vi "Round Timestamp to Tenth of Second.vi"(1 "Time Stamp (now)":timestamp) -> (0 "Time Stamp":timestamp)   [LabVIEW 2011]
doc: "Rounds Timestamp to the nearest tenth of a second.\n\nReturns current time if input is unwired.\n\nVersion 1.0 - 03/07/2013\n\nPhaeron, Inc.\nwww.phaeron.com\ninfo@phaeron.com"
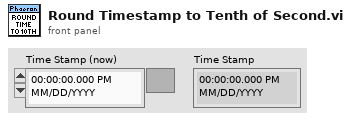
[diagram p1: front panel]
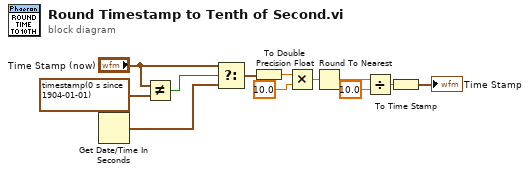
[diagram p0: block diagram]
diagram:
  n1 = Get Date/Time In Seconds() -> (seconds since 1Jan1904=w5:timestamp)
  n2 = Not Equal?(x="Time Stamp (now)", y=timestamp(0 s since 1904-01-01) ("Time Stamp")) -> (x != y?=w4:bool)
  n3 = Select(t="Time Stamp (now)", s=w4, f=w5) -> (s? t:f=w1:timestamp)
  n4 = To Double Precision Float(number=w1) -> (double precision float=w12:dbl)
  n5 = Multiply(x=w12, y=10.0) -> (x*y=w11:dbl)
  n6 = Round To Nearest(number=w11) -> (nearest integer value=w7:dbl)
  n7 = Divide(x=w7, y=10.0) -> (x/y=w9:dbl)
  n8 = To Time Stamp(1:w9) -> (0:→"Time Stamp":timestamp)
